vi "Configure Glitch Capture.vi"(0 "VISA resource name":refnum<visa-resource-name>, 5 "Enable Glitch Capture Display (F: Disable)":bool, 7 "Glitch Capture Display Intensity (50 %)":dbl=50.0, 9 "Foreground Noise Filter Frequency (0: 200 MHz)":u16(ring) items=["200 MHz", "150 MHz", "75 MHz", "42 MHz", "21 MHz", "11 MHz", "5.5 MHz", "2.2 MHz", "1.1 MHz", "550 KHz", "220 KHz", "110 KHz", "55 KHz", "22 KHz", "11 KHz", "5.5 KHz", "2.2 KHz", "1.1 KHz", "550 Hz", "220 Hz", "110 Hz", "55 Hz", "22 Hz", "11 Hz", "1 Hz"], 11 "error in (no error)":errorcluster) -> (4 "VISA resource name out":refnum<visa-resource-name>, 15 "error out":errorcluster)   [LabVIEW 2016, in "Tektronix DPO MSO 2000 4000 Series.lvlib"]
doc: "Configures the FliterVu settings.\n\n<B>Note:</B>\n\nThis VI is only valid for DPO2K and MSO2K series."
uses:
  Tektronix DPO MSO 2000 4000 Series.lvlib
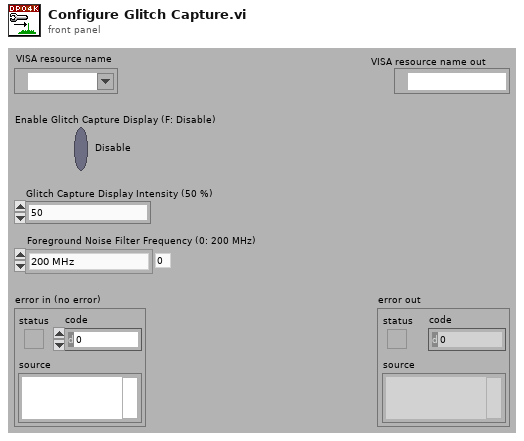
[diagram p1: front panel]
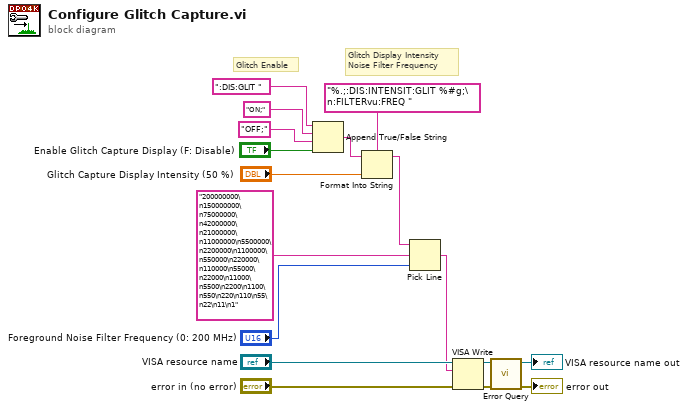
[diagram p0: block diagram]
diagram:
  # "Glitch Display Intensity\nNoise Filter Frequency"
  # "Glitch Enable"
  n1 = Append True/False String(1:"Enable Glitch Capture Display (F: Disable)", 2:"OFF;" ("false string"), 3:"ON;" ("true string"), 4:":DIS:GLIT " ("nkgb.")) -> (0:w5:string)
  n2 = Format Into String(format string="%.;:DIS:INTENSIT:GLIT %#g;\n:FILTERvu:FREQ ", initial string=w5, "Glitch Capture Display Intensity (50 %)") -> (resulting string=w2:string)  [unwired: 1 in, 1 out]
  n3 = Pick Line(string ("")=w2, multi-line string="200000000\n150000000\n75000000\n42000000\n21000000\n11000000\n5500000\n2200000\n1100000\n550000\n220000\n110000\n55000\n22000\n11000\n5500\n2200\n1100\n550\n220\n110\n55\n22\n11\n1", line index="Foreground Noise Filter Frequency (0: 200 MHz)") -> (output string=w1:string)
  n4 = VISA Write(VISA resource name="VISA resource name", write buffer=w1, error in (no error)="error in (no error)") -> (VISA resource name out=w11:refnum<visa-resource-name>, error out=w10:errorcluster)  [unwired: 1 out]
  n5 = call "Error Query.vi"("error in (no error)"=w10, "VISA resource name"=w11) -> ("error out"=→"error out":errorcluster, "VISA resource name out"=→"VISA resource name out":refnum<visa-resource-name>)  [unwired: 6 in, 2 out]
